vi "Configure Trigger External Interface.vi"(0 "VISA resource name":refnum<visa-resource-name>, 1 "Enable Trigger Output (F: Disable)":bool, 5 "Trigger Input Line (1)":u16(ring)=1 items=["1"=1, "2"=2, "3"=3, "4"=4, "5"=5, "6"=6], 7 "Trigger Output Line (2)":u16(ring)=2 items=["1"=1, "2"=2, "3"=3, "4"=4, "5"=5, "6"=6], 11 "error in (no error)":errorcluster) -> (4 "VISA resource name out":refnum<visa-resource-name>, 15 "error out":errorcluster)   [LabVIEW 2020, in "Keithley 648X Series.lvlib"]
doc: "Configures the external trigger interface which deals with the instrument's interaction with other devices."
uses:
  <instrlib>/Keithley 648X Series/Keithley 648X Series.lvlib
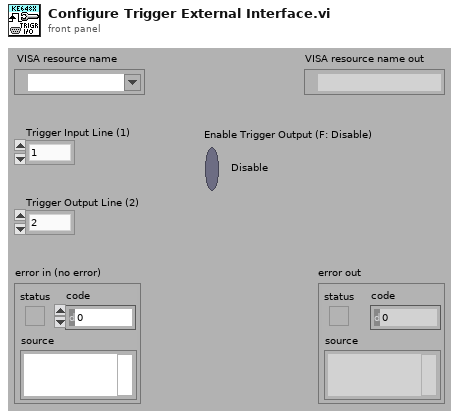
[diagram p1: front panel]
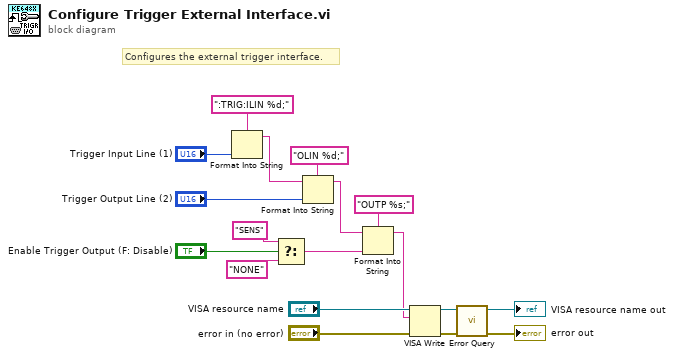
[diagram p0: block diagram]
diagram:
  # "Configures the external trigger interface."
  n1 = Format Into String(format string=":TRIG:ILIN %d;", "Trigger Input Line (1)") -> (resulting string=w2:string)  [unwired: 2 in, 1 out]
  n2 = Select(t="SENS" ("format string"), s="Enable Trigger Output (F: Disable)", f="NONE") -> (s? t:f=w4:string)
  n3 = Format Into String(format string="OLIN %d;", initial string=w2, "Trigger Output Line (2)") -> (resulting string=w3:string)  [unwired: 1 in, 1 out]
  n4 = Format Into String(format string="OUTP %s;", initial string=w3, w4) -> (resulting string=w1:string)  [unwired: 1 in, 1 out]
  n5 = VISA Write(VISA resource name="VISA resource name", write buffer=w1, error in (no error)="error in (no error)") -> (VISA resource name out=w14:refnum<visa-resource-name>, error out=w13:errorcluster)  [unwired: 1 out]
  n6 = call <instrlib>:"Error Query.vi"("error in (no error)"=w13, "VISA resource name"=w14) -> ("error out"=→"error out":errorcluster, "VISA resource name out"=→"VISA resource name out":refnum<visa-resource-name>)  [unwired: 6 in, 2 out]
